vi "demo1_main.vi"() -> ()   [LabVIEW 2016]
uses:
  main/apis/Setup/GetVI/GetVIByPath.vi
  main/apis/Stimulus/ValueSignalByPathString.vi
  <vilib>/addons/_JKI Toolkits/Caraya/classes/Test/Test.lvclass
panel:
  out "error out":errorcluster
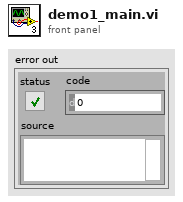
[diagram p1: front panel]
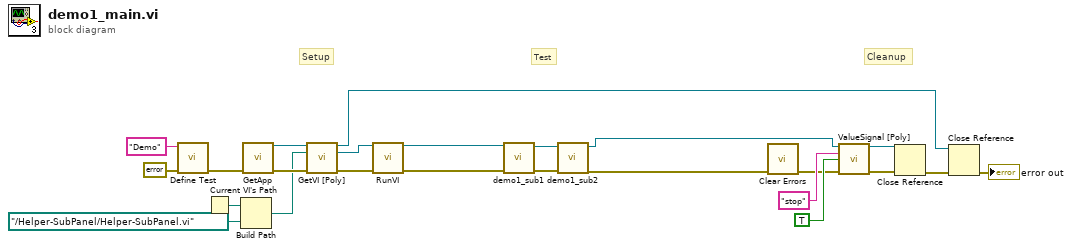
[diagram p0: block diagram]
diagram:
  # "Test"
  # "Cleanup"
  # "Setup"
  n1 = call <vilib>:"Define Test.vi"("error in (no error)"=errorcluster {"status"=FALSE, "code"=0, "source"=""}, "Label (VI Title)"="Demo") -> ("error out"=w23:errorcluster)  [unwired: 9 in]
  n2 = Current VI's Path() -> (path=w16:path)
  n3 = Build Path(base path=w16, name or relative path=path "../Helper-SubPanel/Helper-SubPanel.vi" ("path")) -> (appended path=w17:path)
  n4 = call "GetApp.vi"("error in (no error)"=w23) -> ("Application Ref"=w21:refnum<vi>, "error out"=w20:errorcluster)  [unwired: 13 in]
  n5 = call-poly "GetVI [Poly].vi"("Application Ref in"=w21, "VI Path"=w17, "error in (no error)"=w20) -> ("Application Ref out"=w19:refnum<vi>, "VI Reference"=w13:refnum<vi>, "error out"=w14:errorcluster)  [unwired: 10 in]
  n6 = call "RunVI.vi"("VI Reference In"=w13, "error in"=w14) -> ("VI Reference Out"=w11:refnum<vi>, "error out"=w12:errorcluster)  [unwired: 12 in]
  n7 = call "demo1_sub1.vi"("error in (no error)"=w12, "VI Reference In"=w11) -> ("error out"=w10:errorcluster, "VI Reference Out"=w9:refnum<vi>)  [unwired: 8 in]
  n8 = call "demo1_sub2.vi"("error in (no error)"=w10, "VI Reference In"=w9) -> ("error out"=w4:errorcluster, "VI Reference Out"=w2:refnum<vi>)  [unwired: 8 in]
  n9 = call <vilib>:"Clear Errors.vi"("error in (no error)"=w4) -> ("error out"=w5:errorcluster)  [unwired: 5 in, 1 out]
  n10 = call-poly "ValueSignal [Poly].vi"("VI Reference In"=w2, "Control Name"="stop" ("Class Name"), "Value (Signaling)"=TRUE, "error in"=w5) -> ("VI Reference Out"=w1:refnum<vi>, "error out"=w3:errorcluster)  [unwired: 10 in]
  n11 = Close Reference(reference=w1, error in (no error)=w3) -> (error out=w8:errorcluster)
  n12 = Close Reference(reference=w19, error in (no error)=w8) -> (error out=→"error out":errorcluster)
